vi "Test Complex Operations 1.vi"() -> ()   [LabVIEW 2014]
uses:
  <vilib>/LabVIEW Universal Transcriptor/Arduino for LabVIEW Complex numbers/Complex Numbers.lvlib
panel:
  out "Error Out":errorcluster
  in  "Imag":dbl=-0.78 format="%#_13g"
  in  "Real":dbl=0.22 format="%#_13g"
  in  "Error In":errorcluster
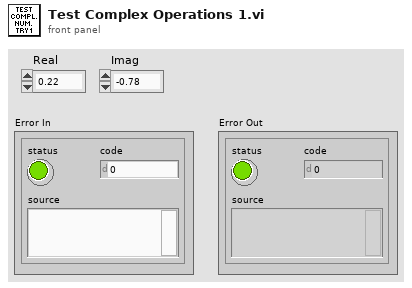
[diagram p1: front panel]
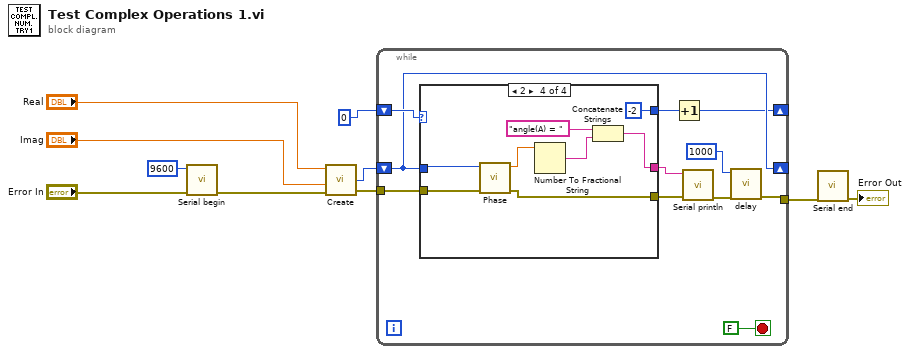
[diagram p0: block diagram]
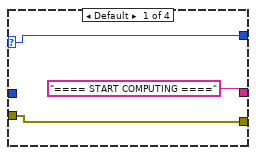
[diagram p2: hidden frame]
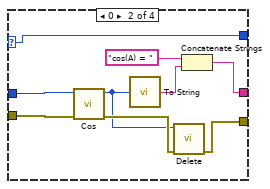
[diagram p3: hidden frame]
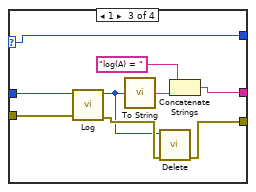
[diagram p4: hidden frame]
diagram:
  n1 = call <vilib>:"Serial begin.vi"("Error In"="Error In", "speed (Bd)"=9600) -> ("Error Out"=w5:errorcluster)  [unwired: 9 in]
  n2 = call <vilib>:"Create.vi"("Error In"=w5, "Imag"="Imag", "Real"="Real") -> ("Error Out"=w8:errorcluster, "Complex"=w7:u32)  [unwired: 2 in]
  n3 = while {
    tunnel: w8 -> [w21]
    tunnel: [w14] -> w2
    shift-right: [w13] -> _
    shift-left: w7 -> [w13]
    shift-right: [w11] -> _
    shift-left: 0 -> [w19]
    stop <- FALSE stop-if-true
    n4 = case shown="2" w19 {
      selector: w19 -> [w22 w28 w37 _]
      tunnel: w21 -> [w24 w33 w42 w50]
      tunnel: w13 -> [_ w29 w41 w44]
      tunnel: [w24 w25 w35 w49] -> w18
      tunnel: ["==== START COMPUTING ====" w30 w39 w46] -> w17
      tunnel: [w22 w28 w37 -2] -> w12
      frame Default {
      }
      frame 0 {
        n5 = call <vilib>:"Cos.vi"("Error In"=w33, "A"=w29) -> ("Error Out"=w27:errorcluster, "sin(A)"=w26:u32)  [unwired: 8 in]
        n6 = call <vilib>:"To String.vi"("Complex number"=w26) -> ("String complex num."=w31:string)
        n7 = call <vilib>:"Delete.vi"("Error In"=w27, "Numeric"=w26) -> ("Error Out"=w25:errorcluster)  [unwired: 9 in]
        n8 = Concatenate Strings("cos(A) = " ("string"), w31) -> (w30:string)
      }
      frame 1 {
        n9 = call <vilib>:"Log.vi"("Error In"=w42, "A"=w41) -> ("Error Out"=w36:errorcluster, "log(A)"=w34:u32)  [unwired: 8 in]
        n10 = call <vilib>:"To String.vi"("Complex number"=w34) -> ("String complex num."=w40:string)
        n11 = call <vilib>:"Delete.vi"("Error In"=w36, "Numeric"=w34) -> ("Error Out"=w35:errorcluster)  [unwired: 9 in]
        n12 = Concatenate Strings("log(A) = " ("string"), w40) -> (w39:string)
      }
      frame 2 {
        n13 = call <vilib>:"Phase.vi"("Error In"=w50, "A"=w44) -> ("Error Out"=w49:errorcluster, "Real part"=w48:dbl)  [unwired: 8 in]
        n14 = Number To Fractional String(number=w48) -> (F-format string=w47:string)  [unwired: 3 in]
        n15 = Concatenate Strings("angle(A) = " ("string"), w47) -> (w46:string)
      }
    }
    n16 = Increment(x=w12) -> (x+1=w11:i32)
    n17 = call <vilib>:"Serial println.vi"("Error In"=w18, "string in"=w17) -> ("Error Out"=w16:errorcluster)  [unwired: 9 in]
    n18 = call <vilib>:"delay.vi"("Error In"=w16, "time (ms)"=1000) -> ("Error Out"=w14:errorcluster)  [unwired: 9 in]
  }
  n19 = call <vilib>:"Serial end.vi"("Error In"=w2) -> ("Error Out"=→"Error Out":errorcluster)  [unwired: 10 in]
